vi "writing to file.vi"() -> ()   [LabVIEW 2009]
doc: "This VI shows how to write data values separated by commas to an ASCII file. The Write Characters To File VI first creates a new file, then appends each value as it is generated."
uses:
  <vilib>/Utility/file.llb/Write To Spreadsheet File (DBL).vi
panel:
  in  "1D data":dbl[](array[numeric]) format="%0.2f"
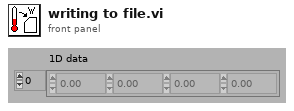
[diagram p1: front panel]
types:
  T1 = enum16{"open", "replace", "create", "open or create", "replace or create", "replace or create with confirmation"}
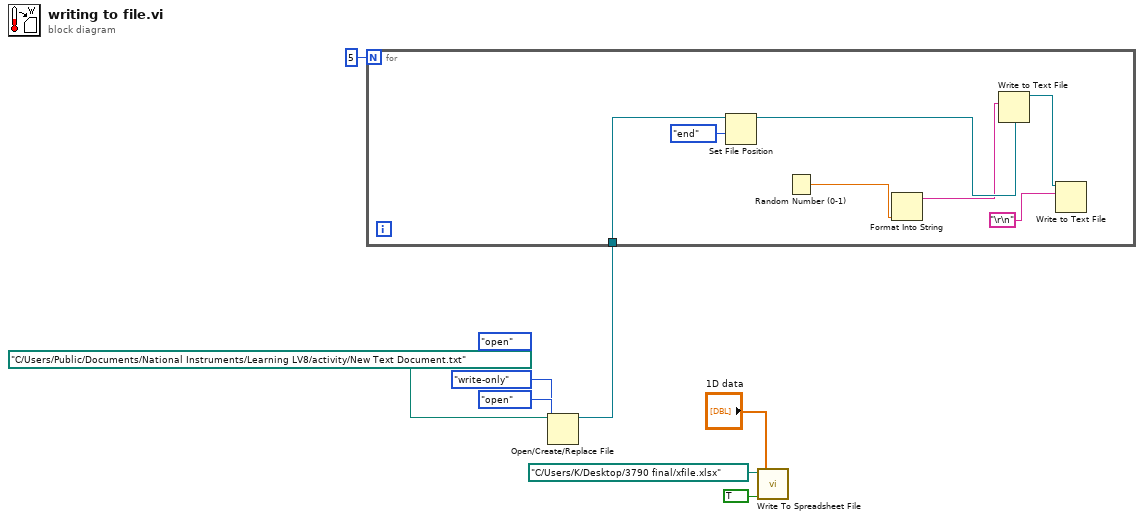
[diagram p0: block diagram]
diagram:
  (unwired) T1."open" ("operation (0:open)")
  n1 = Open/Create/Replace File(file path (use dialog)=path "C:/Users/Public/Documents/National Instruments/Learning LV8/activity/New Text Document.txt", operation (0:open)=T1."open", access (0:read/write)=enum16{"read/write", "read-only", "write-only"}."write-only") -> (refnum out=w4:refnum<file>)  [unwired: 3 in, 2 out]
  n2 = for {
    N: 5 -> [_]
    tunnel: w4 -> [w15]
    n3 = Set File Position(refnum=w15, from (0:start)=enum16{"start", "end", "current"}."end") -> (refnum out=w13:refnum<file>)  [unwired: 2 in, 1 out]
    n4 = Random Number (0-1)() -> (number: 0 to 1=w9:dbl)
    n5 = Format Into String(w9) -> (resulting string=w10:string)  [unwired: 3 in, 1 out]
    n6 = Write to Text File(file (use dialog)=w13, text=w10) -> (refnum out=w12:refnum<file>)  [unwired: 2 in, 2 out]
    n7 = Write to Text File(file (use dialog)=w12, text="\r\n") -> ()  [unwired: 2 in, 3 out]
  }
  n8 = call-poly <vilib>:"Write To Spreadsheet File.vi"("append to file? (new file:F)"=TRUE, "1D data"="1D data", "file path (dialog if empty)"=path "C:/Users/K/Desktop/3790 final/xfile.xlsx") -> ()  [unwired: 5 in, 1 out]
